vi "Color Iterater.vi"(0 "Change Color":bool, 7 "Disable Flash":bool, 13 "Initial Color":T1(ring)) -> (4 "Color":T1(ring), 8 "Display Mode":T2(ring))   [LabVIEW 2016]
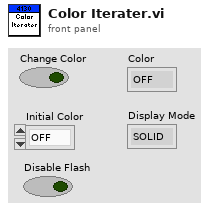
[diagram p1: front panel]
types:
  T1 = enum16{"OFF", "RED", "GREEN", "BLUE", "PURPLE", "YELLOW", "TEAL", "WHITE", "RAINBOW"}
  T2 = enum16{"SOLID", "FLASH 500ms", "FLASH 1000ms", "OFF"}
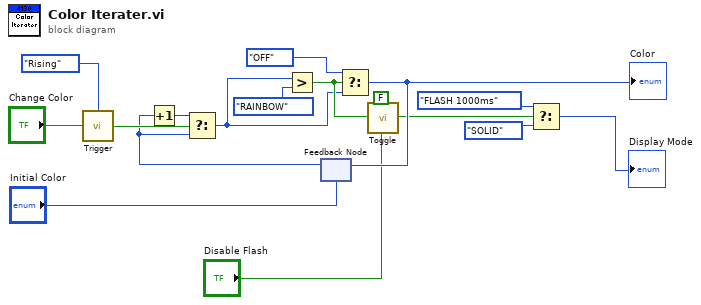
[diagram p0: block diagram]
diagram:
  n1 = call "Trigger.vi"("Enum"=enum16{"Falling", "Rising", "Both"}."Rising", "Button"="Change Color") -> ("Trigger"=w5:bool)  [unwired: 13 in]
  n2 = feedback #1("Initial Color") -> (w1:T1)
  n3 = Increment(x=w1) -> (x+1=w7:T1)
  n4 = Select(t=w7, s=w5, f=w1) -> (s? t:f=w9:T1)
  n5 = Greater?(x=w9, y=T1."RAINBOW" ("lower limit")) -> (0:w11:bool)
  n6 = Select(t=T1."OFF" ("lower limit"), s=w11, f=w9) -> (s? t:f=w17:T1)
  "Color" <- w17
  n7 = feedback-in #1(w17) -> ()
  n8 = call "Toggle.vi"("Trigger"=w11, "Initialize (F)"=FALSE, "Override to initialize value"="Disable Flash") -> ("Output"=w12:bool)  [unwired: 24 in]
  n9 = Select(t=T2."FLASH 1000ms" ("Display Mode"), s=w12, f=T2."SOLID" ("Display Mode")) -> (s? t:f=→"Display Mode":T2)
